vi "Make Movement Proposals.vi"(0 "Elves in":set{T1}(c389), 1 "Movement Proposal Rules":T2(array[cluster])) -> (2 "Elves' Movement Proposals":map{T1, T1}(c390))   [LabVIEW 2020, in "AoC 2022.lvlib"]
uses:
  AoC 2022.lvlib
  Day 15 - Beacon Exclusion Zone/private/Location.ctl
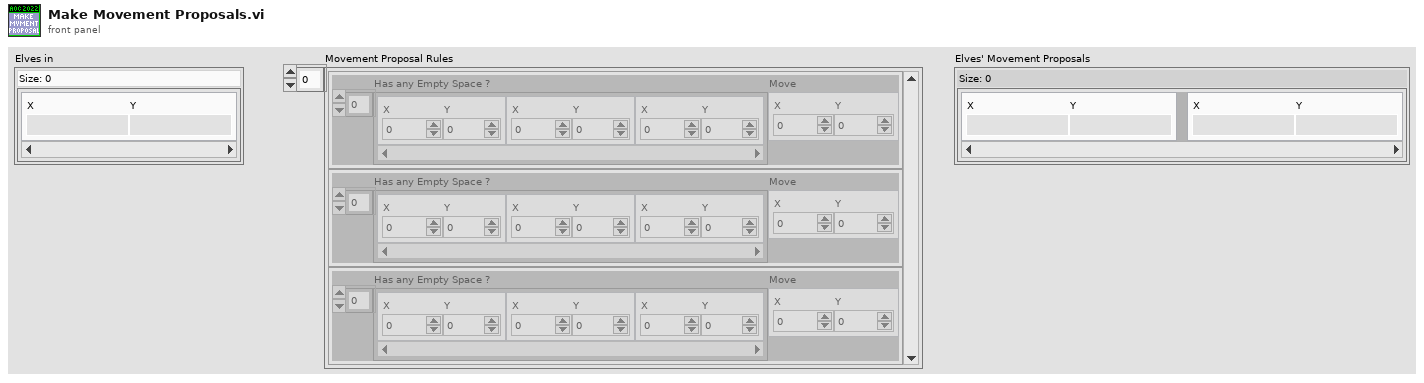
[diagram p1: front panel]
types:
  T1 = typedef "AoC 2022.lvlib/Location.ctl" = cluster{"X":i32, "Y":i32}
  T2 = cluster{"Has any Empty Space ?":T1[], "Move":T1}[]
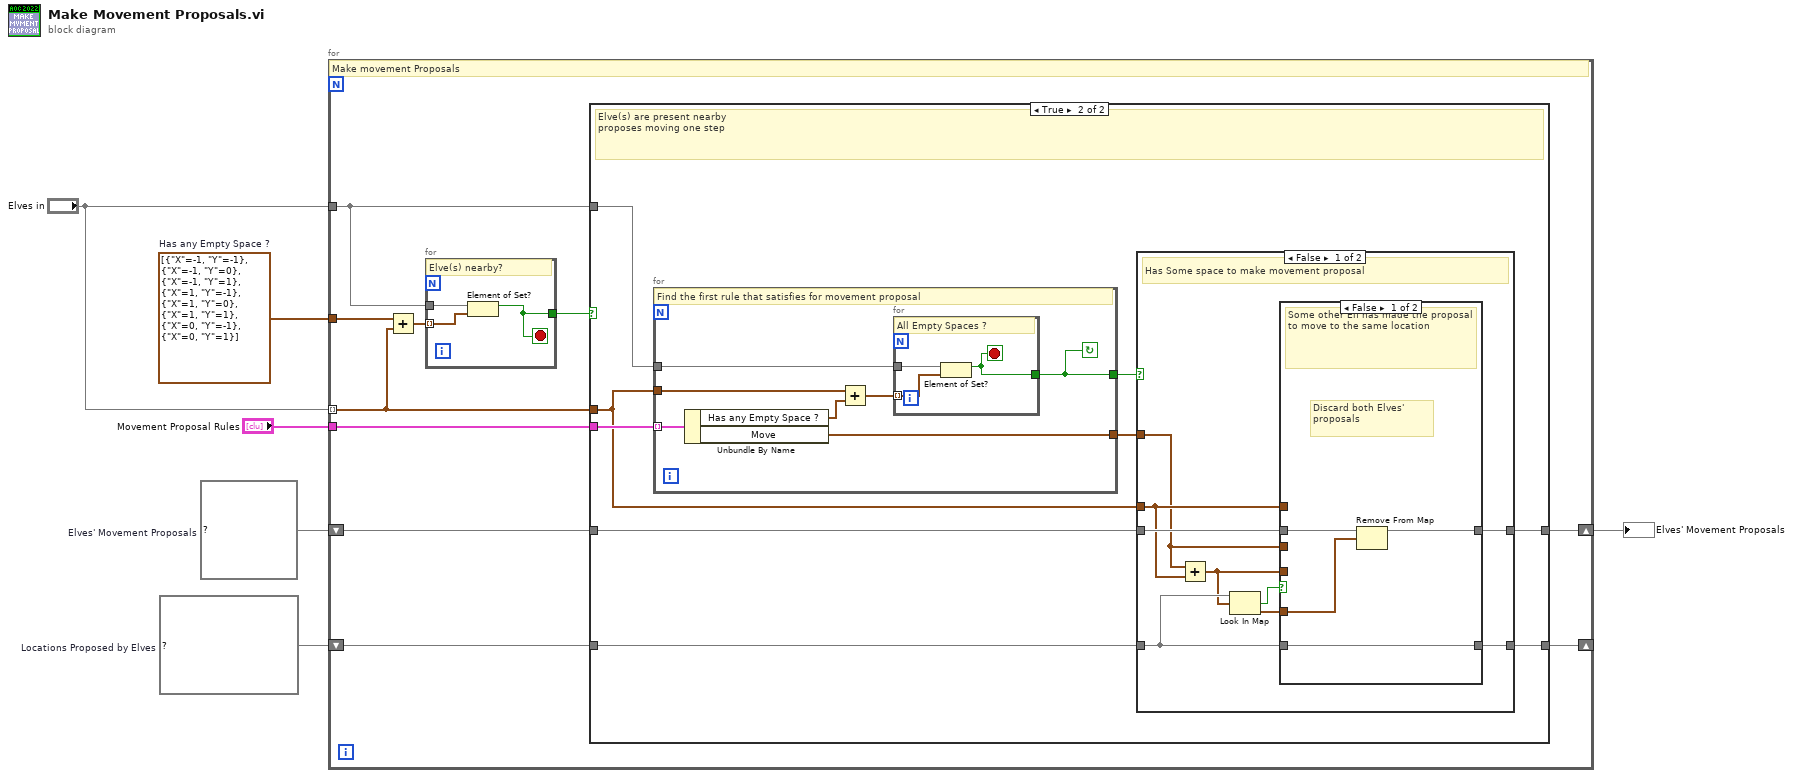
[diagram p0: block diagram]
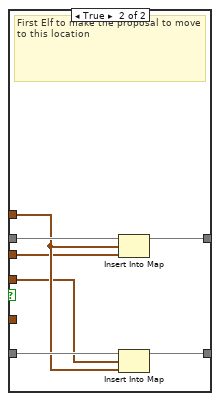
[diagram p3: hidden frame]
diagram:
  w6 = map{T1, T1} {}  # Locations Proposed by Elves
  w5 = map{T1, T1} {}  # Elves' Movement Proposals
  w4 = T1[] [{"X"=-1, "Y"=-1}, {"X"=-1, "Y"=0}, {"X"=-1, "Y"=1}, {"X"=1, "Y"=-1}, {"X"=1, "Y"=0}, {"X"=1, "Y"=1}, {"X"=0, "Y"=-1}, {"X"=0, "Y"=1}]  # Has any Empty Space ?
  n1 = for {
    tunnel: "Elves in" -> [w8] mode=indexing
    tunnel: w4 -> [w16]
    shift-right: [w13] -> _
    shift-left: w6 -> [w12]
    shift-right: [w11] -> w1
    shift-left: w5 -> [w10]
    tunnel: "Elves in" -> [w7]
    tunnel: "Movement Proposal Rules" -> [w9]
    # "Make movement Proposals"
    n2 = Add(x=w16, y=w8) -> (x+y=w15:T1[])
    n3 = for {
      tunnel: w15 -> [w61] mode=indexing
      tunnel: w7 -> [w62]
      tunnel: [w60] -> w14
      stop <- w60 stop-if-true
      # "Elve(s) nearby?"
      n4 = Element of Set?(10:w61, 11:w62) -> (3:w60:bool)
    }
    n5 = case shown="True" w14 {
      tunnel: w9 -> [_ w27]
      tunnel: [w18 w22] -> w13
      tunnel: w12 -> [w18 w24]
      tunnel: [w17 w23] -> w11
      tunnel: w10 -> [w17 w25]
      tunnel: w8 -> [_ w20]
      tunnel: w7 -> [_ w19]
      frame False {
        # "No Elves are present nearby\ndoes not do anything"
      }
      frame True {
        # "Elve(s) are present nearby\nproposes moving one step"
        n6 = for {
          tunnel: w27 -> [w56] mode=indexing
          tunnel: w20 -> [w54]
          tunnel: w19 -> [w53]
          tunnel: [w51] -> w26
          tunnel: [w50] -> w21
          stop <- w51 continue-if-true
          # "Find the first rule that satisfies for movement proposal"
          n7 = Unbundle By Name(w56) -> ("Has any Empty Space ?"=w55:T1[], "Move"=w50:T1)
          n8 = Add(x=w54, y=w55) -> (x+y=w52:T1[])
          n9 = for {
            tunnel: w53 -> [w59]
            tunnel: w52 -> [w58] mode=indexing
            tunnel: [w57] -> w51
            stop <- w57 stop-if-true
            # "All Empty Spaces ?"
            n10 = Element of Set?(10:w58, 11:w59) -> (3:w57:bool)
          }
        }
        n11 = case shown="False" w26 {
          tunnel: w25 -> [w35 w49]
          tunnel: w24 -> [w32 w48]
          tunnel: [w36 w49] -> w23
          tunnel: [w34 w48] -> w22
          tunnel: w21 -> [w29 _]
          tunnel: w20 -> [w30 _]
          frame False {
            # "Has Some space to make movement proposal"
            n12 = Add(x=w29, y=w30) -> (x+y=w28:T1)
            n13 = Look In Map(map=w32, key=w28) -> (key not found?=w33:bool, value=w31:T1)  [unwired: 1 in]
            n14 = case shown="False" w33 {
              tunnel: w32 -> [w40 w45]
              tunnel: [w39 w46] -> w36
              tunnel: w35 -> [w38 w47]
              tunnel: [w40 w44] -> w34
              tunnel: w30 -> [_ w43]
              tunnel: w29 -> [_ w42]
              tunnel: w31 -> [w37 _]
              tunnel: w28 -> [_ w41]
              frame False {
                # "Discard both Elves' proposals"
                # "Some other Elf has made the proposal to move to the same location"
                n15 = Remove From Map(10:w37, 11:w38) -> (3:w39:map{T1, T1})  [unwired: 2 out]
              }
              frame True {
                # "First Elf to make the proposal to move to this location"
                n16 = Insert Into Map(map in=w47, key=w43, value=w42) -> (map out=w46:map{T1, T1})  [unwired: 2 out]
                n17 = Insert Into Map(map in=w45, key=w41, value=w43) -> (map out=w44:map{T1, T1})  [unwired: 2 out]
              }
            }
          }
          frame True {
            # "No Valid Directions to propose for movement"
          }
        }
      }
    }
  }
  "Elves' Movement Proposals" <- w1
